vi "Main.vi"(11 "Module Admin":refnum<class "Delacor_lib_QMH_Module Admin.lvclass">) -> ()   [LabVIEW 2019, in "UI.lvlib"]
doc: "This template is based off of the Queued Message Handler design pattern and the Queued Message Handler project template that ships with LabVIEW.\n\nThe main difference is that the queue is private to this module and communication between modules is performed via Broadcast and Request events.\n\nRequest events are wrapped in public API methods and are handled in the Event Handling Loop (EHL) of this VI. Any module can register for Broadcast events sent by this module. The EHL generates messages based on user interface actions.\n\nThe Message Handling Loop (MHL) processes messages generated by the EHL, or by other messages. The messages are string values, so new messages can be added easily to the Message Cases case structure in the MHL. Each message cluster can also provide an optional value for Message Data, which is a variant that can be converted to whatever message-specific data is required.\n_____\nBased on DQMH Project Template 6.1.0.94."
uses:
  UI.lvlib
  <vilib>/Delacor/Delacor QMH/Libraries/Module Admin_class/Delacor_lib_QMH_Module Admin.lvclass
  Module Data--cluster.ctl
  Do Something Argument--cluster.ctl
  <vilib>/Delacor/Delacor QMH/Libraries/Message Queue_class/Delacor_lib_QMH_Message Queue.lvclass/Delacor_lib_QMH_Message Queue.ctl
  Do Something Else Argument--cluster.ctl
  Do Something Else and Wait for Reply Argument--cluster.ctl
  Do Something Else and Wait (Reply Payload)--cluster.ctl
  Stop Argument--cluster.ctl
  <vilib>/Delacor/Delacor QMH/Libraries/Module Admin_class/Delacor_lib_QMH_Module Admin.lvclass/Delacor_lib_QMH_Module Admin.ctl
  <vilib>/Utility/miscctls.llb/LVPointTypeDef.ctl
  <vilib>/Delacor/Delacor QMH/Libraries/Message Queue_class/Delacor_lib_QMH_Enqueue Message (Single).vi
  <vilib>/Delacor/Delacor QMH/Libraries/Module Admin_class/Delacor_lib_QMH_Get External Launch.vi
  <vilib>/Utility/error.llb/Error Cluster From Error Code.vi
  <vilib>/ErrorRing/Error Ring.xnode
  <vilib>/Delacor/Delacor QMH/Libraries/Message Queue_class/Delacor_lib_QMH_Message Queue.lvclass
panel:
  out "error out":errorcluster
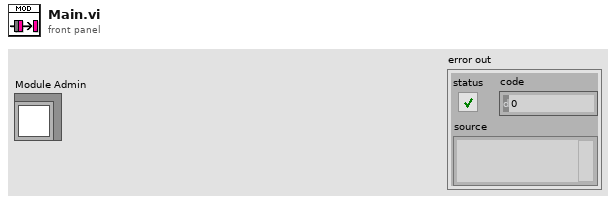
[diagram p1: front panel]
types:
  T1 = typedef "UI.lvlib/Request Events--cluster.ctl" = cluster{"Stop Module":refnum<user-event>, "Do Something":refnum<user-event>, "Do Something Else":refnum<user-event>, "Do Something Else and Wait for Reply":refnum<user-event>, "Show Panel":refnum<user-event>, "Hide Panel":refnum<user-event>, "Get Module Execution Status":refnum<user-event>, "Show Diagram":refnum<user-event>}
  T2 = typedef "UI.lvlib/Module Data--cluster.ctl" = cluster{"Status":string}
  T3 = typedef "UI.lvlib/Do Something Argument--cluster.ctl" = cluster{"Do Something Msg":string}
  T4 = typedef "UI.lvlib/Do Something Else Argument--cluster.ctl" = cluster{"Do Something Else Msg":string, "X":dbl}
  T5 = typedef "UI.lvlib/Do Something Else and Wait for Reply Argument--cluster.ctl" = cluster{"Do Something Else Msg":string, "X":dbl, "Wait Notifier":refnum<notifier>, "wait for reply":bool}
  T6 = enum32{"invalid lock state", "Not Locked", "Locked (No Password)", "Password-protected"}
  T7 = typedef "UI.lvlib/Stop Argument--cluster.ctl" = cluster{"Origin":string, "Exit via Stop Module Req?":bool, "Wait for Module to stop?":bool}
  T8 = typedef "LVPointTypeDef.ctl" = cluster{"Horizontal":i16, "Vertical":i16}
  T9 = enum32{"Invalid", "Standard", "Closed", "Hidden", "Minimized", "Maximized"}
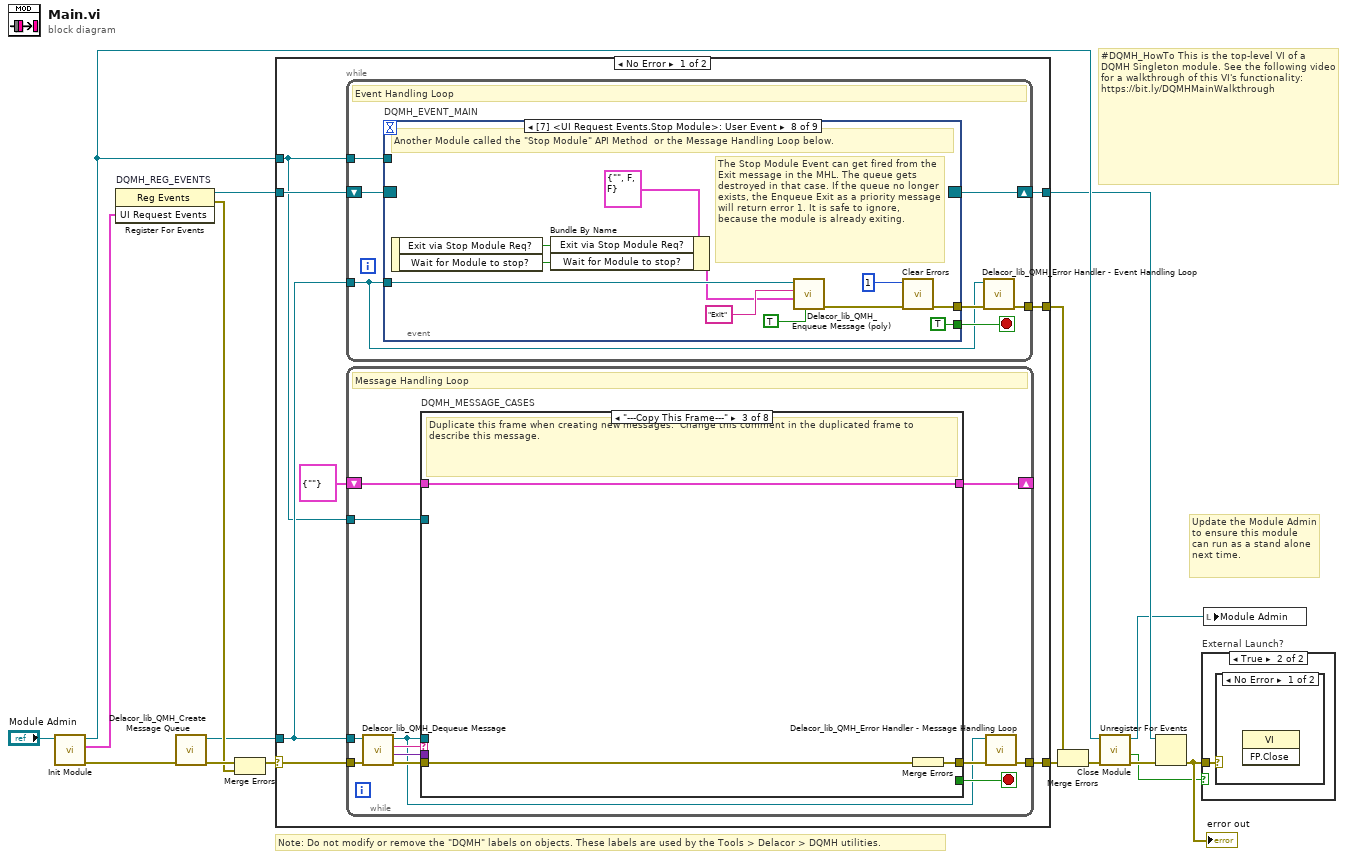
[diagram p0: block diagram]
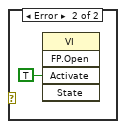
[diagram p3: hidden frame]
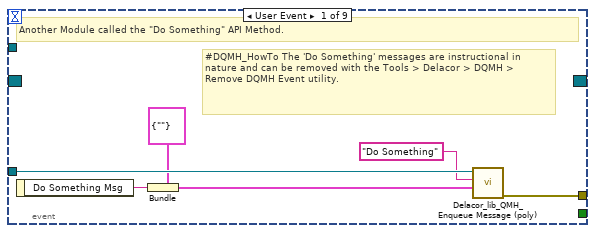
[diagram p4: hidden frame]
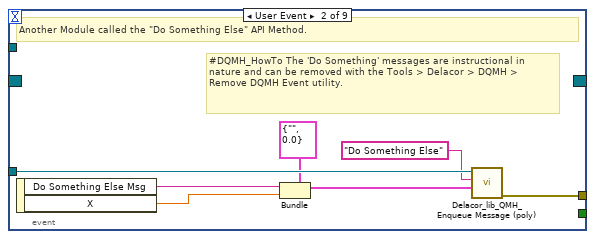
[diagram p5: hidden frame]
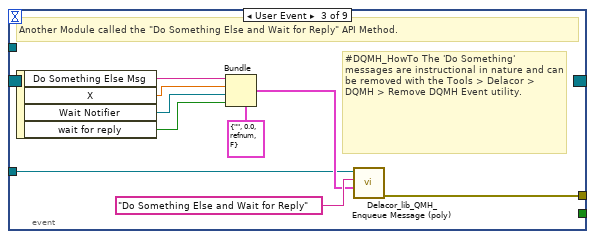
[diagram p6: hidden frame]
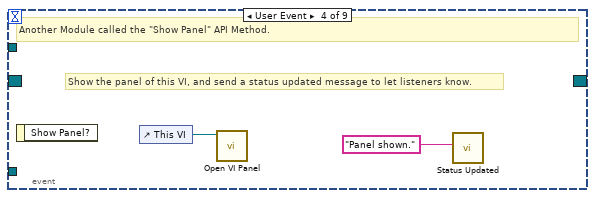
[diagram p7: hidden frame]
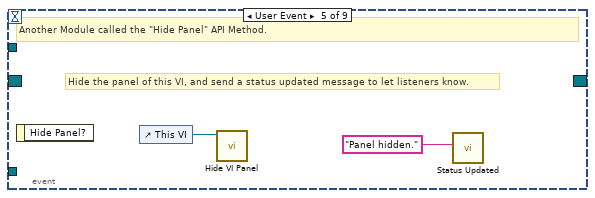
[diagram p8: hidden frame]
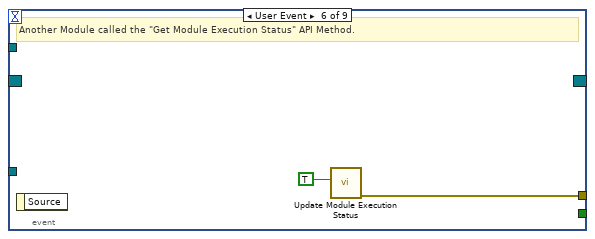
[diagram p9: hidden frame]
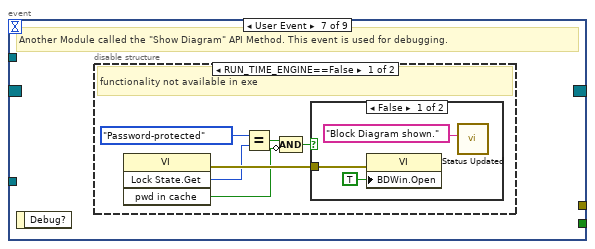
[diagram p10: hidden frame]
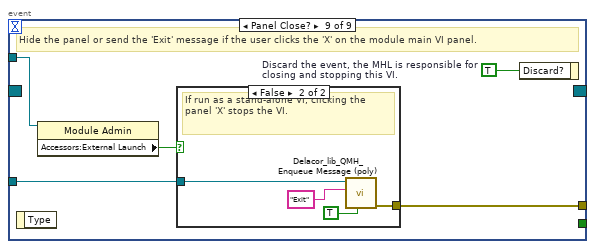
[diagram p13: hidden frame]
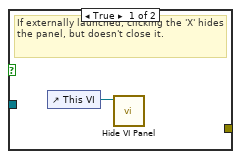
[diagram p14: hidden frame]
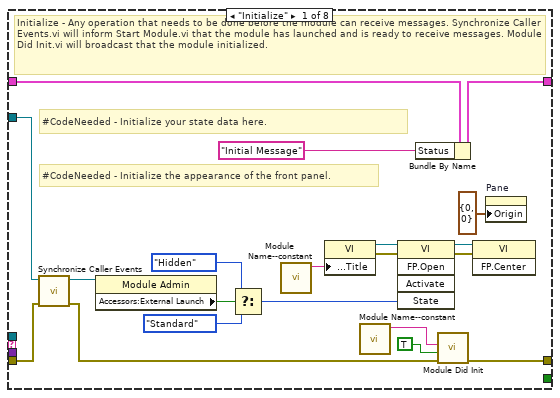
[diagram p15: hidden frame]
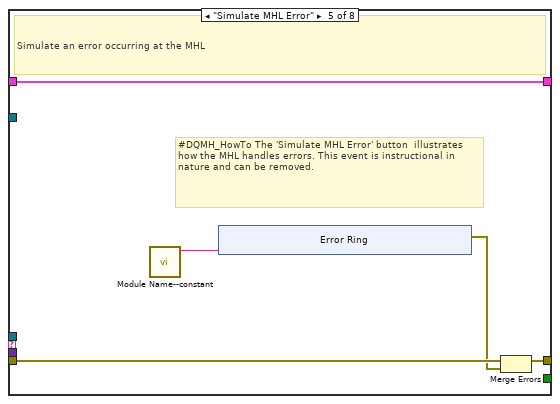
[diagram p18: hidden frame]
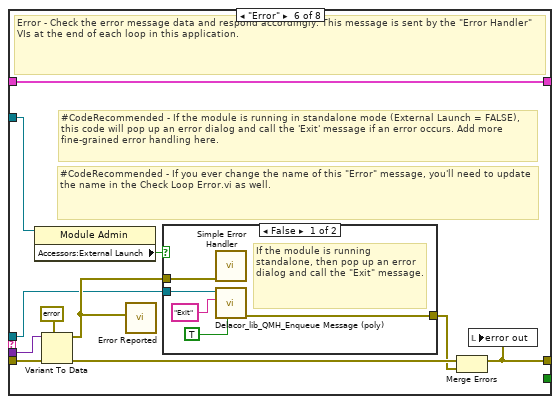
[diagram p19: hidden frame]
diagram:
  # "#DQMH_HowTo This is the top-level VI of a DQMH Singleton module. See the following video for a walkthrough of this VI's functionality: https://bit.ly/DQMHMainWalkthrough"
  # "Note: Do not modify or remove the \"DQMH\" labels on objects. These labels are used by the Tools > Delacor > DQMH utilities."
  # "Update the Module Admin to ensure this module can run as a stand alone next time."
  n1 = call "Init Module.vi"("Singleton Module Admin in"="Module Admin") -> ("error out"=w16:errorcluster, "UI Request Events"=w5:T1, "Singleton Module Admin out"=w8:refnum<class "Delacor_lib_QMH_Module Admin.lvclass">)  [unwired: 8 in]
  n2 = register-events "DQMH_REG_EVENTS"(w5) -> (reference out=w6:refnum<event-registration>, error out=w9:errorcluster)  [unwired: 2 in]
  n3 = call <vilib>:"Delacor_lib_QMH_Create Message Queue.vi"("error in"=w16) -> ("error out"=w11:errorcluster, "Message Queue"=w4:refnum<class "Delacor_lib_QMH_Message Queue.lvclass">)  [unwired: 9 in]
  n4 = Merge Errors(w11, w9) -> (w10:errorcluster)
  n5 = case shown="No Error" w10 {
    selector: w10 -> [w23 w189]
    tunnel: [w25 w188] -> w17
    tunnel: [w22 w194] -> w7
    tunnel: w6 -> [w20 w194]
    tunnel: w4 -> [w19 w187]
    tunnel: [w24 _] -> w14
    tunnel: w8 -> [w18 w190]
    frame No Error {
      n6 = while {
        tunnel: w19 -> [w26]
        shift-right: [w29] -> w22
        shift-left: w20 -> [w30]
        tunnel: [w31] -> w24
        tunnel: w18 -> [w27]
        stop <- w28 stop-if-true
        # "Event Handling Loop"
        n7 = event "DQMH_EVENT_MAIN" shown="[7] <UI Request Events.Stop Module>: User Event" {
          selector: w30 -> [_ _ _ _ _ _ _ _ _]
          dyn-events: [_ _ _ _ _ _ _ _ _] -> w29
          timeout: _ -> [_ _ _ _ _ _ _ _ _]
          tunnel: [_ _ _ _ _ _ _ TRUE ("Discard?") _] -> w28
          tunnel: w26 -> [w37 w44 w47 _ _ _ _ w76 w83]
          tunnel: [w38 w45 w54 _ _ w60 _ w79 w85] -> w32
          tunnel: w27 -> [_ _ _ _ _ _ _ _ w82]
          event User Event {
            # "#DQMH_HowTo The 'Do Something' messages are instructional in nature and can be removed with the Tools > Delacor > DQMH > Remove DQMH Event utility."
            # "Another Module called the \"Do Something\" API Method."
            n8 = event-data() -> ("Do Something Msg"=w34:string)  [unwired: 1 in]
            n9 = Bundle(cluster=T3 {"Do Something Msg"=""} ("Do Something Argument"), "Do Something Msg"=w34) -> (w33:T3)
            n10 = call-poly <vilib>:"Delacor_lib_QMH_Enqueue Message (poly).vi"("Message Data"=w33, "Message"="Do Something", "Message Queue in"=w37) -> ("error out"=w38:errorcluster)  [unwired: 7 in, 1 out]
          }
          event User Event {
            # "#DQMH_HowTo The 'Do Something' messages are instructional in nature and can be removed with the Tools > Delacor > DQMH > Remove DQMH Event utility."
            # "Another Module called the \"Do Something Else\" API Method."
            n11 = event-data() -> ("Do Something Else Msg"=w40:string, "X"=w39:dbl)  [unwired: 1 in]
            n12 = Bundle(cluster=T4 {"Do Something Else Msg"="", "X"=0.0} ("Do Something Else Argument"), "Do Something Else Msg"=w40, "X"=w39) -> (w41:T4)
            n13 = call-poly <vilib>:"Delacor_lib_QMH_Enqueue Message (poly).vi"("Message Data"=w41, "Message"="Do Something Else", "Message Queue in"=w44) -> ("error out"=w45:errorcluster)  [unwired: 7 in, 1 out]
          }
          event User Event {
            # "#DQMH_HowTo The 'Do Something' messages are instructional in nature and can be removed with the Tools > Delacor > DQMH > Remove DQMH Event utility."
            # "Another Module called the \"Do Something Else and Wait for Reply\" API Method."
            n14 = event-data() -> ("Do Something Else Msg"=w50:string, "X"=w49:dbl, "Wait Notifier"=w48:refnum<notifier>, "wait for reply"=w46:bool)  [unwired: 1 in]
            n15 = Bundle(cluster=T5 {"Do Something Else Msg"="", "X"=0.0, "Wait Notifier"=refnum, "wait for reply"=FALSE} ("Do Something Else and Wait for Reply Argument"), "Do Something Else Msg"=w50, "X"=w49, "Wait Notifier"=w48, "wait for reply"=w46) -> (w51:T5)
            n16 = call-poly <vilib>:"Delacor_lib_QMH_Enqueue Message (poly).vi"("Message Data"=w51, "Message"="Do Something Else and Wait for Reply", "Message Queue in"=w47) -> ("error out"=w54:errorcluster)  [unwired: 7 in, 1 out]
          }
          event User Event {
            # "Show the panel of this VI, and send a status updated message to let listeners know."
            # "Another Module called the \"Show Panel\" API Method."
            n17 = event-data() -> ()  [unwired: 1 in, 1 out]
            n18 = control-ref of="This VI"() -> (w56:refnum<vi>)
            n19 = call "Open VI Panel.vi"("VI"=w56) -> ()  [unwired: 10 in, 1 out]
            n20 = call "Status Updated.vi"("Status"="Panel shown." ("format string")) -> ()  [unwired: 10 in, 1 out]
          }
          event User Event {
            # "Hide the panel of this VI, and send a status updated message to let listeners know."
            # "Another Module called the \"Hide Panel\" API Method."
            n21 = event-data() -> ()  [unwired: 1 in, 1 out]
            n22 = control-ref of="This VI"() -> (w58:refnum<vi>)
            n23 = call "Hide VI Panel.vi"("VI"=w58) -> ()  [unwired: 10 in, 1 out]
            n24 = call "Status Updated.vi"("Status"="Panel hidden." ("format string")) -> ()  [unwired: 10 in, 1 out]
          }
          event User Event {
            # "Another Module called the \"Get Module Execution Status\" API Method."
            n25 = event-data() -> ()  [unwired: 1 in, 1 out]
            n26 = call "Update Module Execution Status.vi"("Running?"=TRUE) -> ("error out"=w60:errorcluster)  [unwired: 10 in]
          }
          event User Event {
            # "Another Module called the \"Show Diagram\" API Method. This event is used for debugging."
            n27 = event-data() -> ()  [unwired: 1 in, 1 out]
            n28 = disable-structure shown="RUN_TIME_ENGINE==False" {
              frame condition #0 (active) {
                # "functionality not available in exe"
                n29 = invoke class="VI" method="Lock State.Get"() -> (error out=w66:errorcluster, "Get Lock State"=w65:T6, "pwd in cache"=w62:bool)  [unwired: 4 in, 1 out]
                n30 = Equal?(x=T6."Password-protected", y=w65) -> (x = y?=w63:bool)
                n31 = Compound Arithmetic op=AND(w63, invert w62) -> (w61:bool)
                n32 = case shown="False" w61 {
                  tunnel: w66 -> [w69 _]
                  frame False {
                    n33 = property class="VI"(error in=w69, "BDWin.Open"=TRUE ("Block Diagram Window:Open")) -> ()  [unwired: 1 in, 2 out]
                    n34 = call "Status Updated.vi"("Status"="Block Diagram shown." ("format string")) -> ()  [unwired: 10 in, 1 out]
                  }
                  frame True {
                    # "Password-protected VI, and the password is not in the cache. Do not show the diagram."
                  }
                }
              }
              frame condition #1 {
              }
            }
          }
          event User Event {
            # "The Stop Module Event can get fired from the Exit message in the MHL. The queue gets destroyed in that case. If the queue no longer exists, the Enqueue Exit as a priority message will return error 1. It is safe to ignore, because the module is already exiting."
            # "Another Module called the \"Stop Module\" API Method  or the Message Handling Loop below."
            n35 = event-data() -> ("Exit via Stop Module Req?"=w72:bool, "Wait for Module to stop?"=w71:bool)  [unwired: 1 in]
            n36 = Bundle By Name(cluster=T7 {"Origin"="", "Exit via Stop Module Req?"=FALSE, "Wait for Module to stop?"=FALSE} ("Stop Argument"), "Exit via Stop Module Req?"=w72, "Wait for Module to stop?"=w71) -> (w70:T7)
            n37 = call-poly <vilib>:"Delacor_lib_QMH_Enqueue Message (poly).vi"("Priority Message? (F)"=TRUE, "Message Data"=w70, "Message"="Exit", "Message Queue in"=w76) -> ("error out"=w80:errorcluster)  [unwired: 6 in, 1 out]
            n38 = call <vilib>:"Clear Errors.vi"("error in (no error)"=w80, "specific error code to clear (0: all)"=1) -> ("error out"=w79:errorcluster)  [unwired: 4 in, 1 out]
          }
          event Panel Close? {
            w84 = TRUE  # Discard the event, the MHL is responsible for closing and stopping this VI.
            # "Hide the panel or send the 'Exit' message if the user clicks the 'X' on the module main VI panel."
            n39 = event-data() -> ()  [unwired: 1 in, 1 out]
            n40 = property class="Module Admin"(reference=w82) -> ("Accessors:External Launch"=w81:bool)  [unwired: 1 in, 2 out]
            n41 = case shown="False" w81 {
              tunnel: w83 -> [_ w89]
              tunnel: [_ w90] -> w85
              frame True {
                # "If externally launched, clicking the 'X' hides the panel, but doesn't close it."
                n42 = control-ref of="This VI"() -> (w86:refnum<vi>)
                n43 = call "Hide VI Panel.vi"("VI"=w86) -> ()  [unwired: 10 in, 1 out]
              }
              frame False {
                # "If run as a stand-alone VI, clicking the panel 'X' stops the VI."
                n44 = call-poly <vilib>:"Delacor_lib_QMH_Enqueue Message (poly).vi"("Priority Message? (F)"=TRUE, "Message"="Exit", "Message Queue in"=w89) -> ("error out"=w90:errorcluster)  [unwired: 7 in, 1 out]
              }
            }
            n45 = event-data("Discard?"=w84) -> ()  [unwired: 1 in, 1 out]
          }
        }
        n46 = call-dynamic "Delacor_lib_QMH_Error Handler - Event Handling Loop.vi"("error in"=w32, "Message Queue in"=w26) -> ("dup error in"=w31:errorcluster)  [unwired: 8 in, 1 out]
      }
      n47 = while {
        tunnel: w19 -> [w93]
        shift-right: [w97] -> _
        shift-left: T2 {"Status"=""} ("Data Cluster") -> [w98]
        tunnel: w23 -> [w101]
        tunnel: [w99] -> w25
        tunnel: w18 -> [w91]
        stop <- w96 stop-if-true
        # "Message Handling Loop"
        n48 = call-dynamic "Delacor_lib_QMH_Dequeue Message.vi"("error in"=w101, "Message Queue in"=w93) -> ("error out"=w100:errorcluster, "Message Data"=w94:variant, "Message"=w95:string, "Message Queue out"=w92:refnum<class "Delacor_lib_QMH_Message Queue.lvclass">)  [unwired: 6 in]
        n49 = case "DQMH_MESSAGE_CASES" shown="\"---Copy This Frame---\"" w95 {
          selector: w95 -> [_ _ _ _ _ _ _ w174]
          tunnel: w92 -> [_ _ _ _ _ w144 w166 _]
          tunnel: w100 -> [w120 w124 w127 w129 w134 w151 w172 w176]
          tunnel: [w118 w124 w126 w129 w133 w147 w169 w177] -> w102
          tunnel: w98 -> [w109 w123 w125 w128 w131 w146 w165 w175]
          tunnel: [w108 w123 w125 w128 w131 w146 w165 w175] -> w97
          tunnel: [_ _ _ _ _ _ w164 _] -> w96
          tunnel: w94 -> [_ _ _ _ _ w145 w163 _]
          tunnel: w91 -> [w110 _ _ _ _ w143 w158 _]
          frame "Initialize" {
            # "#CodeNeeded - Initialize the appearance of the front panel."
            # "#CodeNeeded - Initialize your state data here."
            # "Initialize - Any operation that needs to be done before the module can receive messages. Synchronize Caller Events.vi will inform Start Module.vi that the module has launched and is ready to receive messages. Module Did Init.vi will broadcast that the module initialized."
            n50 = call "Synchronize Caller Events.vi"("error in (no error)"=w120, "Singleton Module Admin in"=w110) -> ("error out"=w119:errorcluster, "Singleton Module Admin out"=w105:refnum<class "Delacor_lib_QMH_Module Admin.lvclass">)  [unwired: 8 in]
            n51 = property class="Module Admin"(reference=w105) -> ("Accessors:External Launch"=w114:bool)  [unwired: 1 in, 2 out]
            n52 = Select(t=T9."Hidden" ("State"), s=w114, f=T9."Standard" ("State")) -> (s? t:f=w111:T9)
            n53 = call "Module Name--constant.vi"() -> ("Module Name"=w117:string)  [unwired: 11 in]
            n54 = property class="VI"("Front Panel.Title"=w117) -> (reference out=w116:refnum<vi>, error out=w122:errorcluster)  [unwired: 2 in]
            n55 = call "Module Name--constant.vi"() -> ("Module Name"=w106:string)  [unwired: 11 in]
            n56 = invoke class="VI" method="FP.Open"(reference=w116, error in=w122, "State"=w111) -> (reference out=w115:refnum<vi>, error out=w121:errorcluster)  [unwired: 2 in, 3 out]
            n57 = Bundle By Name(cluster=w109, "Status"="Initial Message" ("Initial Message")) -> (w108:T2)
            n58 = call "Module Did Init.vi"("error in (no error)"=w119, "Initialized?"=TRUE, "Origin"=w106) -> ("error out"=w118:errorcluster)  [unwired: 8 in]
            n59 = invoke class="VI" method="FP.Center"(reference=w115, error in=w121) -> ()  [unwired: 1 in, 3 out]
            n60 = property on="Pane" class="Pane"("Origin"=T8 {"Horizontal"=0, "Vertical"=0}) -> ()  [unwired: 2 in, 2 out]
          }
          frame "---Module Specific---" {
            # "Separator -- The following cases handle messages specific to this Module."
          }
          frame "---Copy This Frame---" {
            # "Duplicate this frame when creating new messages.  Change this comment in the duplicated frame to describe this message."
            n61 = Merge Errors(w127) -> (w126:errorcluster)
          }
          frame "---Exit and Error Handling---" {
            # "Separator - The following cases handle errors and exit messages."
          }
          frame "Simulate MHL Error" {
            # "#DQMH_HowTo The 'Simulate MHL Error' button  illustrates how the MHL handles errors. This event is instructional in nature and can be removed."
            # "Simulate an error occurring at the MHL"
            n62 = call "Module Name--constant.vi"() -> ("Module Name"=w130:string)  [unwired: 11 in]
            n63 = xnode "Error Ring"("parameter 0"=w130) -> ("error out"=w132:errorcluster)
            n64 = Merge Errors(w134, w132) -> (w133:errorcluster)
          }
          frame "Error" {
            # "#CodeRecommended - If you ever change the name of this \"Error\" message, you'll need to update the name in the Check Loop Error.vi as well."
            # "#CodeRecommended - If the module is running in standalone mode (External Launch = FALSE), this code will pop up an error dialog and call the 'Exit' message if an error occurs. Add more fine-grained error handling here."
            # "Error - Check the error message data and respond accordingly. This message is sent by the \"Error Handler\" VIs at the end of each loop in this application."
            n65 = property class="Module Admin"(reference=w143) -> ("Accessors:External Launch"=w142:bool)  [unwired: 1 in, 2 out]
            n66 = Variant To Data(error in=w151, type=errorcluster {"status"=FALSE, "code"=0, "source"=""} ("error constant"), Variant=w145) -> (data=w152:errorcluster, error out=w149:errorcluster)
            n67 = call "Error Reported.vi"("Error"=w152) -> ()  [unwired: 10 in, 1 out]
            n68 = case shown="False" w142 {
              tunnel: [w157 _] -> w148
              tunnel: w144 -> [w155 _]
              tunnel: w152 -> [w156 _]
              frame False {
                # "If the module is running standalone, then pop up an error dialog and call the \"Exit\" message."
                n69 = call <vilib>:"Simple Error Handler.vi"("error in (no error)"=w156) -> ()  [unwired: 4 in, 5 out]
                n70 = call-poly <vilib>:"Delacor_lib_QMH_Enqueue Message (poly).vi"("Priority Message? (F)"=TRUE, "Message"="Exit", "Message Queue in"=w155) -> ("error out"=w157:errorcluster)  [unwired: 7 in, 1 out]
              }
              frame True {
                # "If the module was launched externally, calling the Error Reported broadcast VI is the only action performed by the \"Error\" message. The module's caller can then process the error appropriately."
              }
            }
            n71 = Merge Errors(w149, w148) -> (w147:errorcluster)
            n72 = local write "error out"(w147) -> ()
          }
          frame "Exit" {
            w162 = 91  # 91: not all Exit messages will have an argument
            w164 = TRUE  # Stop the VI
            # "Release the message queue reference"
            # "#CodeNeeded - Add any required cleanup code here"
            # "Exit - Exit the application."
            n73 = Variant To Data(error in=w172, type=T7 {"Origin"="", "Exit via Stop Module Req?"=FALSE, "Wait for Module to stop?"=FALSE} ("Stop Argument"), Variant=w163) -> (data=w160:T7, error out=w168:errorcluster)
            n74 = call <vilib>:"Clear Errors.vi"("error in (no error)"=w168, "specific error code to clear (0: all)"=w162) -> ("error out"=w171:errorcluster)  [unwired: 4 in, 1 out]
            n75 = control-ref of="This VI"() -> (w159:refnum<vi>)
            n76 = call-dynamic "Delacor_lib_QMH_Release Message Queue.vi"("error in"=w171, "Message Queue"=w166) -> ("error out"=w170:errorcluster)  [unwired: 9 in]
            n77 = call "Handle Exit.vi"("Stop Argument"=w160, "Admin in"=w158, "VI reference"=w159) -> ("error out"=w167:errorcluster)  [unwired: 7 in, 1 out]
            n78 = Merge Errors(w170, w167) -> (w169:errorcluster)
          }
          frame Default {
            # "'Default' case only runs if there is a message that isn't defined in any of the other cases.  Output a programming error."
            n79 = call "Module Name--constant.vi"() -> ("Module Name"=w173:string)  [unwired: 11 in]
            n80 = xnode "Error Ring"("parameter 0"=w174, "parameter 1"=w173) -> ("error out"=w178:errorcluster)
            n81 = Merge Errors(w176, w178) -> (w177:errorcluster)
          }
        }
        n82 = call-dynamic "Delacor_lib_QMH_Error Handler - Message Handling Loop.vi"("error in"=w102, "Message Queue in"=w92) -> ("dup error in"=w99:errorcluster)  [unwired: 8 in, 1 out]
      }
    }
    frame Error {
      # "Synchronize Caller Events.vi will inform Start Module.vi that the module has launched and will let the code calling Start Module.vi register for broadcasts and would permit the caller receive the broadcast that an error occurred at launch time."
      n83 = call-dynamic "Delacor_lib_QMH_Release Message Queue.vi"("error in"=w189, "Message Queue"=w187) -> ("error out"=w188:errorcluster)  [unwired: 9 in]
      n84 = call "Synchronize Caller Events.vi"("Singleton Module Admin in"=w190) -> ("error out"=w195:errorcluster)  [unwired: 9 in, 1 out]
      n85 = call "Module Name--constant.vi"() -> ("Module Name"=w193:string)  [unwired: 11 in]
      n86 = Format Into String(format string="An error occurred during initialization. %s is no longer running.", w193) -> (resulting string=w191:string)  [unwired: 2 in, 1 out]
      n87 = Merge Errors(w188, w195) -> (w196:errorcluster)
      n88 = call "Error Reported.vi"("Additional Information"=w191, "Error"=w196) -> ()  [unwired: 9 in, 1 out]
    }
  }
  n89 = Merge Errors(w14, w17) -> (w13:errorcluster)
  n90 = call "Close Module.vi"("error in (no error)"=w13, "Module Admin in"=w8) -> ("error out"=w15:errorcluster, "External Launch"=w1:bool, "Module Admin out"=w2:refnum<class "Delacor_lib_QMH_Module Admin.lvclass">)  [unwired: 7 in]
  n91 = Unregister For Events(event registration refnum=w7, error in=w15) -> (error out=w12:errorcluster)
  "error out" <- w12
  n92 = case "External Launch?" shown="True" w1 {
    tunnel: w12 -> [_ w197]
    frame False {
    }
    frame True {
      n93 = case shown="No Error" w197 {
        frame No Error {
          n94 = invoke class="VI" method="FP.Close"() -> ()  [unwired: 3 in, 3 out]
        }
        frame Error {
          n95 = invoke class="VI" method="FP.Open"("Activate"=TRUE ("Activate?")) -> ()  [unwired: 4 in, 5 out]
        }
      }
    }
  }
  n96 = local write "Module Admin"(w2) -> ()
